vi "Delete Elements From Array - boolean.vi"(8 "indices (none)":i32[](array[numeric])=[3, 5], 11 "1D Array":bool[](array[boolean])) -> (0 "deleted elements":bool[](array[boolean]), 3 "array w/ subset deleted":bool[](array[boolean]))   [LabVIEW 2020]
doc: "Deletes elements from 1-dim array and returns the edited array in array w/ subset deleted and the deleted elements in deleted portion. A list-based version of the built-in \"Delete From Array\". Note that the \"array with subset deleted\" is returned in a different order than the original array."
uses:
  Index Array Elements/Index Array Elements - boolean.vi
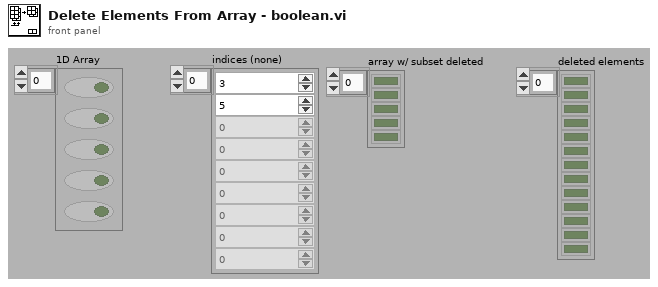
[diagram p1: front panel]
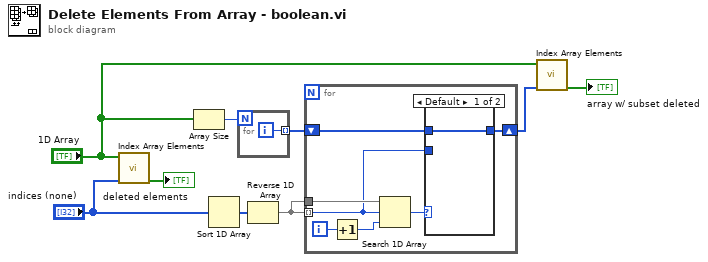
[diagram p0: block diagram]
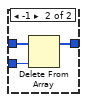
[diagram p2: hidden frame]
diagram:
  n1 = call-poly "Index Array Elements.vi"("indices (none)"="indices (none)", "1D Array"="1D Array") -> ("output array"=→"deleted elements":bool[])  [unwired: 5 in]
  n2 = Array Size(array="1D Array") -> (size(s)=w6:i32)
  n3 = Sort 1D Array(array="indices (none)") -> (sorted array=w5:i32[])
  n4 = for {
    N: w6 -> [_]
    tunnel: [w10] -> w3 mode=indexing
    i -> [w10]
  }
  n5 = Reverse 1D Array(array=w5) -> (reversed array=w1:i32[])
  n6 = for {
    tunnel: w1 -> [w11] mode=indexing
    shift-right: [w16] -> w2
    shift-left: w3 -> [w17]
    tunnel: w1 -> [w15]
    i -> [w13]
    n7 = Increment(x=w13) -> (x+1=w12:i32)
    n8 = Search 1D Array(1D array=w15, element=w11, start index (0)=w12) -> (index of element=w14:i32)
    n9 = case shown="Default" w14 {
      tunnel: w17 -> [w18 w21]
      tunnel: [w18 w20] -> w16
      tunnel: w11 -> [_ w19]
      frame Default {
      }
      frame -1 {
        n10 = Delete From Array(array=w21, index=w19) -> (array with subset deleted=w20:i32[])  [unwired: 1 in, 1 out]
      }
    }
  }
  n11 = call-poly "Index Array Elements.vi"("indices (none)"=w2, "1D Array"="1D Array") -> ("output array"=→"array w/ subset deleted":bool[])  [unwired: 5 in]
